vi "IsOddDBL.vi"(4 "x":dbl) -> (1 "Odd?":bool)   [LabVIEW 2017, in "GPComparison.lvlib"]
doc: "<B>Odd?</B> will be True if <B>x</B> is an odd integer.\n\nThis VI is inlined.\n\nSteen Schmidt\nGPower\n6/3 2013"
uses:
  GPComparison.lvlib
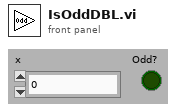
[diagram p1: front panel]
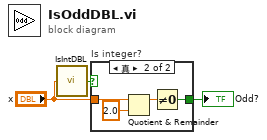
[diagram p0: block diagram]
diagram:
  n1 = call "IsIntDBL.vi"("x"="x") -> ("Integer?"=w2:bool)  [unwired: 4 in]
  n2 = case "Is integer?" shown="真" w2 {
    tunnel: [_ w4] -> w3
    tunnel: "x" -> [_ w7]
    frame False {
    }
    frame True {
      n3 = Quotient & Remainder(x=w7, y=2.0) -> (x-y*floor(x/y)=w5:dbl)  [unwired: 1 out]
      n4 = Not Equal To 0?(x=w5) -> (x != 0?=w4:bool)
    }
  }
  "Odd?" <- w3
